vi "Start Sweep.vi"(7 "Channel (1)":i32=1, 8 "error in (no error)":errorcluster, 11 "VISA resource name":refnum<visa-resource-name>) -> (0 "error out":errorcluster, 3 "VISA resource name out":refnum<visa-resource-name>)   [LabVIEW 2012, in "Tektronix TTR500 Series.lvlib"]
doc: "Changes the state of each channel of selected channel to the startup state in the trigger system.\n\nWhen this function is executed for a channel in the idle state, it goes into the initiate state immediately. Then, after measurement is executed once, it goes back to the idle state.\n\nIf this function is executed for a channel that is not in the idle state or for which the continuous initiation mode is enabled, an error occurs."
uses:
  <instrlib>/Tektronix TTR500 Series/Tektronix TTR500 Series.lvlib
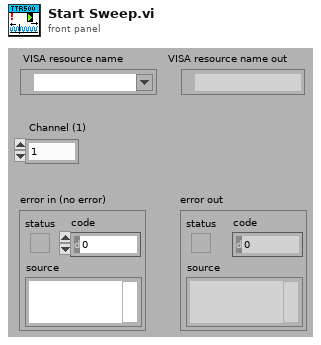
[diagram p1: front panel]
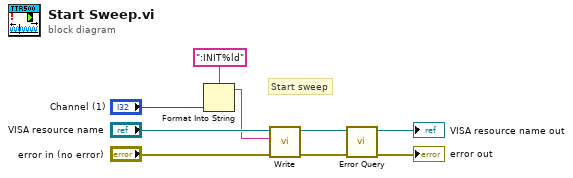
[diagram p0: block diagram]
diagram:
  # "Start sweep"
  n1 = Format Into String(format string=":INIT%ld", "Channel (1)") -> (resulting string=w5:string)  [unwired: 2 in, 1 out]
  n2 = call <instrlib>:"Write.vi"("error in (no error)"="error in (no error)", "String ()"=w5, "VISA resource name"="VISA resource name") -> ("error out"=w3:errorcluster, "VISA resource name out"=w4:refnum<visa-resource-name>)  [unwired: 6 in, 1 out]
  n3 = call <instrlib>:"Error Query.vi"("error in (no error)"=w3, "VISA resource name"=w4) -> ("error out"=→"error out":errorcluster, "VISA resource name out"=→"VISA resource name out":refnum<visa-resource-name>)  [unwired: 6 in, 2 out]
